vi "DB and DP to RH.vi"(1 "Dew Point [DegF]":dbl=50.0, 2 "Dry Bulb Temp [DegF]":dbl=78.0) -> (0 "Relative Humidity [%]":dbl=1.392554657511521)   [LabVIEW 2020]
panel:
  in  "a":dbl=-4.9283
  in  "b1":dbl=-5287.32
  in  "b":dbl=-5287.32
  in  "c1":dbl=23.2801
  in  "c":dbl=23.2801
  in  "a1":dbl=-4.9283
  in  "d":dbl=459.4
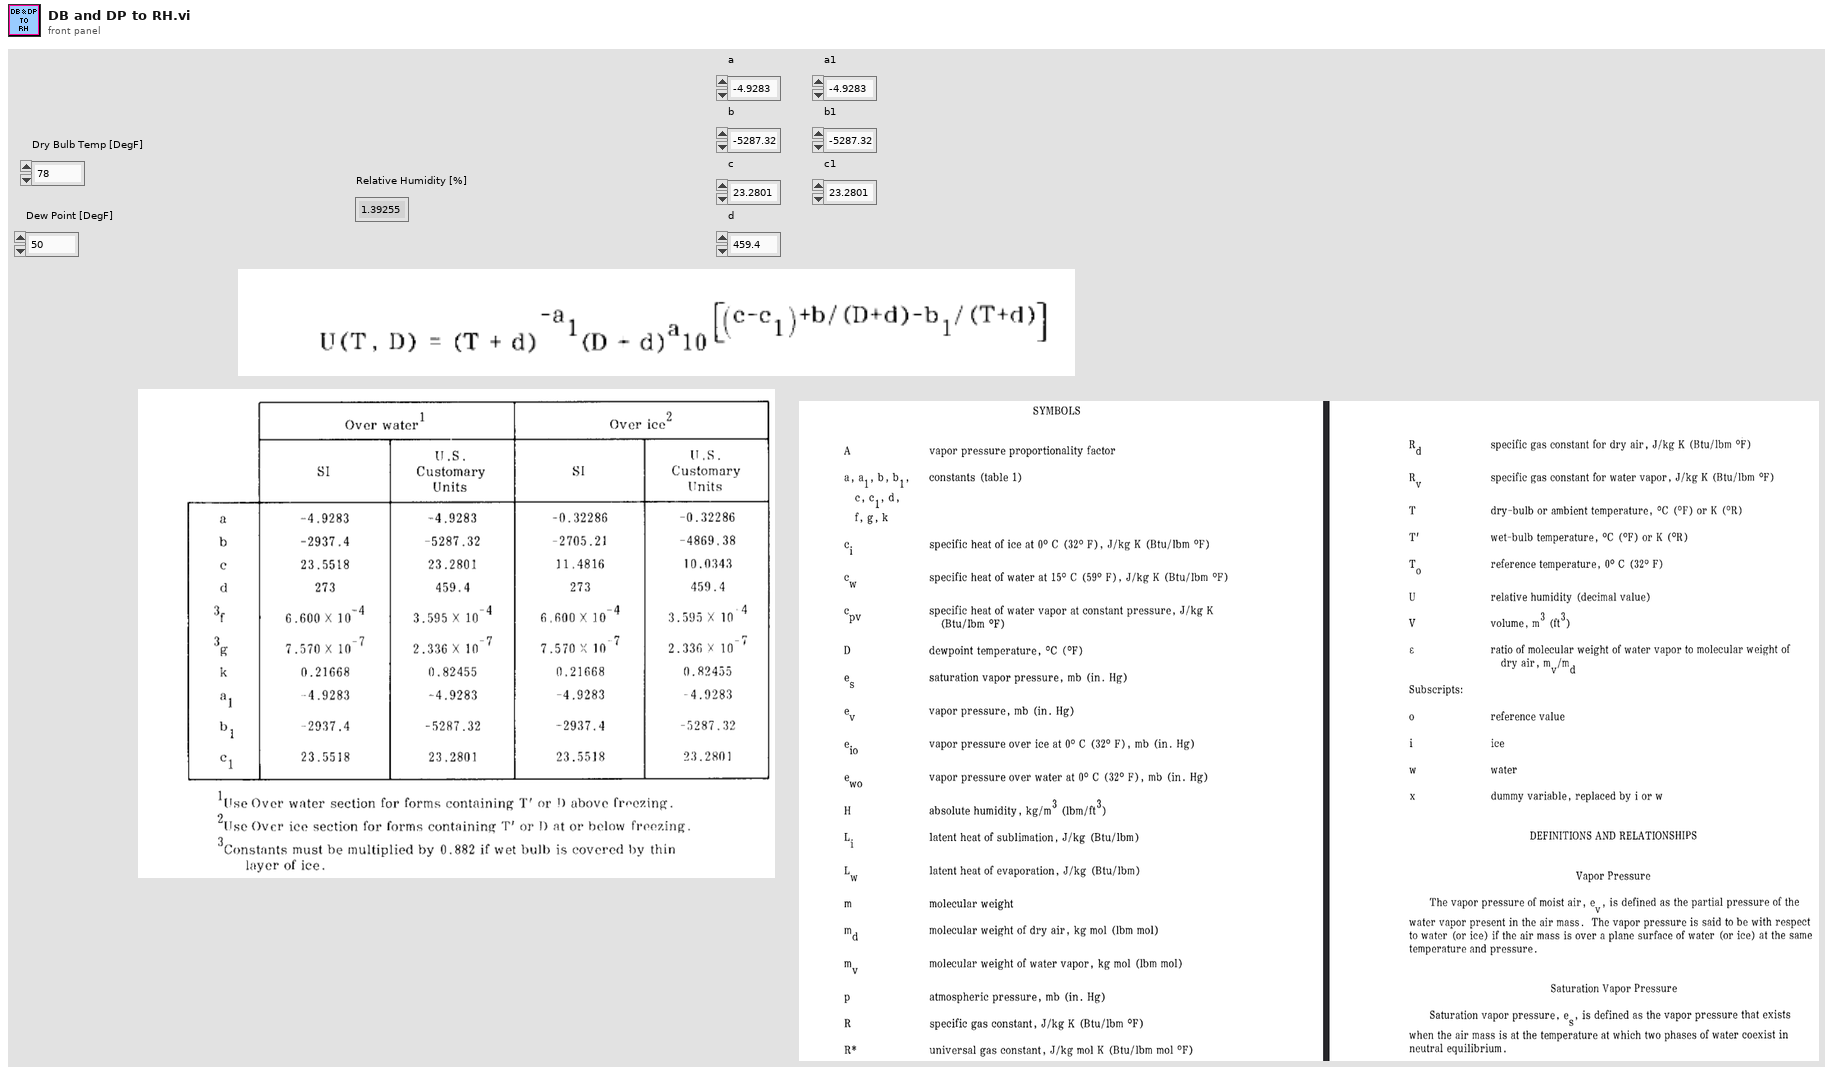
[diagram p1: front panel]
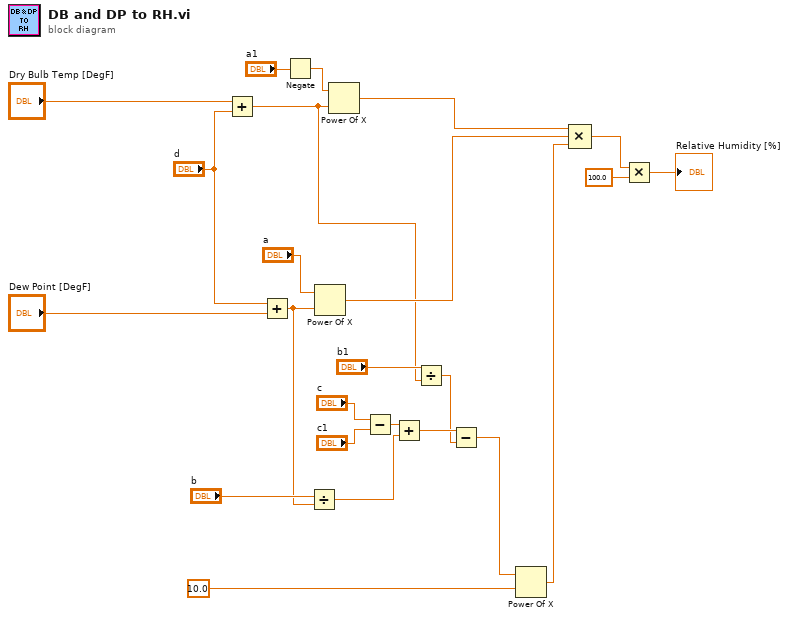
[diagram p0: block diagram]
diagram:
  n1 = Add(x="Dry Bulb Temp [DegF]", y="d") -> (x+y=w7:dbl)
  n2 = Add(x="d", y="Dew Point [DegF]") -> (x+y=w11:dbl)
  n3 = Negate(x="a1") -> (-x=w22:dbl)
  n4 = Divide(x="b", y=w11) -> (x/y=w10:dbl)
  n5 = Power Of X(1:w11, 2:"a") -> (0:w17:dbl)
  n6 = Power Of X(1:w7, 2:w22) -> (0:w21:dbl)
  n7 = Subtract(x="c", y="c1") -> (x-y=w13:dbl)
  n8 = Add(x=w13, y=w10) -> (x+y=w9:dbl)
  n9 = Divide(x="b1", y=w7) -> (x/y=w6:dbl)
  n10 = Subtract(x=w9, y=w6) -> (x-y=w5:dbl)
  n11 = Power Of X(1:10.0, 2:w5) -> (0:w4:dbl)
  n12 = Compound Arithmetic op=MULTIPLY(w21, w17, w4) -> (w2:dbl)
  n13 = Multiply(x=w2, y=100.0) -> (x*y=→"Relative Humidity [%]":dbl)
